vi "QTrkReadJPEGFile.vi"(11 "Path":path) -> (3 "Image":u8[][](array[numeric]))   [LabVIEW 2011]
uses:
  QTrkDLL.vi
panel:
  in  "Image":u8[][](array[numeric])
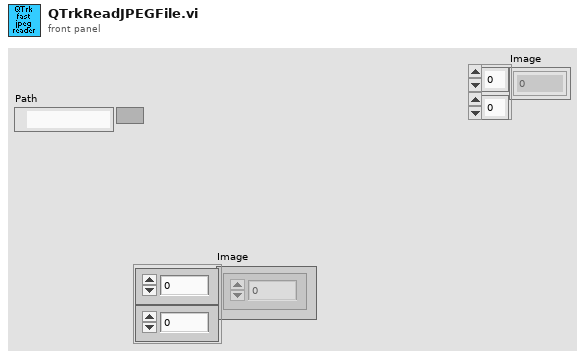
[diagram p1: front panel]
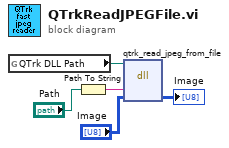
[diagram p0: block diagram]
diagram:
  n1 = global read "QTrkDLL.vi" "QTrk DLL Path"() -> (w3:path)
  n2 = Path To String(path="Path") -> (string=w1:string)
  n3 = dll-call lib="D:/jcnossen1/cudaqi-tracker/bin/jtrkd-labview.dll" fn="qtrk_read_jpeg_from_file"(path in=w3, "filename"=w1, "outputArray"="Image") -> ("outputArray"=→"Image":u8[][])  [unwired: 4 in, 2 out]
